vi "JSON Config Update Test Cases.vi"() -> ()   [LabVIEW 2021]
uses:
  OOB_Rx/CIFCoreOOB_Rx.lvclass/CIFCoreOOB_Rx.ctl
  <vilib>/CIF Foundation/CIF Out of Band Commands/CIFOutOfBand.lvclass/CIFOutOfBand.ctl
  OOB_Rx/Private/Command Settings.vi
  <vilib>/CIF Foundation/CIF Out of Band Commands/Accessors/Write Local OOB Data.vi
  <vilib>/CIF Foundation/CIF Out of Band Commands/Accessors/Read Local OOB Data.vi
  <vilib>/CIF Foundation/CIF Out of Band Commands/Read Commands.vi
  OOB_Rx/Private/Read Payload.vi
  <vilib>/CIF Foundation/CIF Out of Band Commands/Queue Command.vi
  <vilib>/CIF Foundation/CIF Out of Band Commands/Utilities/Command to Bitwise Command.vi
  OOB_Rx/CIFCoreOOB_Rx.lvclass
  C:/Program Files/National Instruments/LabVIEW 2021/vi.lib/CIF Foundation/CIF Out of Band Commands/CIFOutOfBand.lvclass
  <vilib>/CIF Foundation/CIF Out of Band Commands/Init OOB.vi
  <vilib>/addons/_JKI.lib/Serialization/JSON/Library/Unflatten From JSON String.vi
  <vilib>/addons/_JKI.lib/Serialization/JSON/JKI JSON Serialization.lvlib
  <vilib>/CIF Foundation/CIF Out of Band Commands/CIFOutOfBand.lvclass
panel:
  out "pass":bool
  out "error out":errorcluster
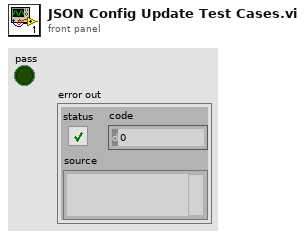
[diagram p1: front panel]
types:
  T1 = cluster{"Numeric":dbl, "String":string, "Boolean":bool}[]
  T2 = cluster{"Numeric":dbl, "Array":cluster{"Numeric":dbl, "String":string, "Boolean":bool}[], "string":string, "Null array":u8[]}
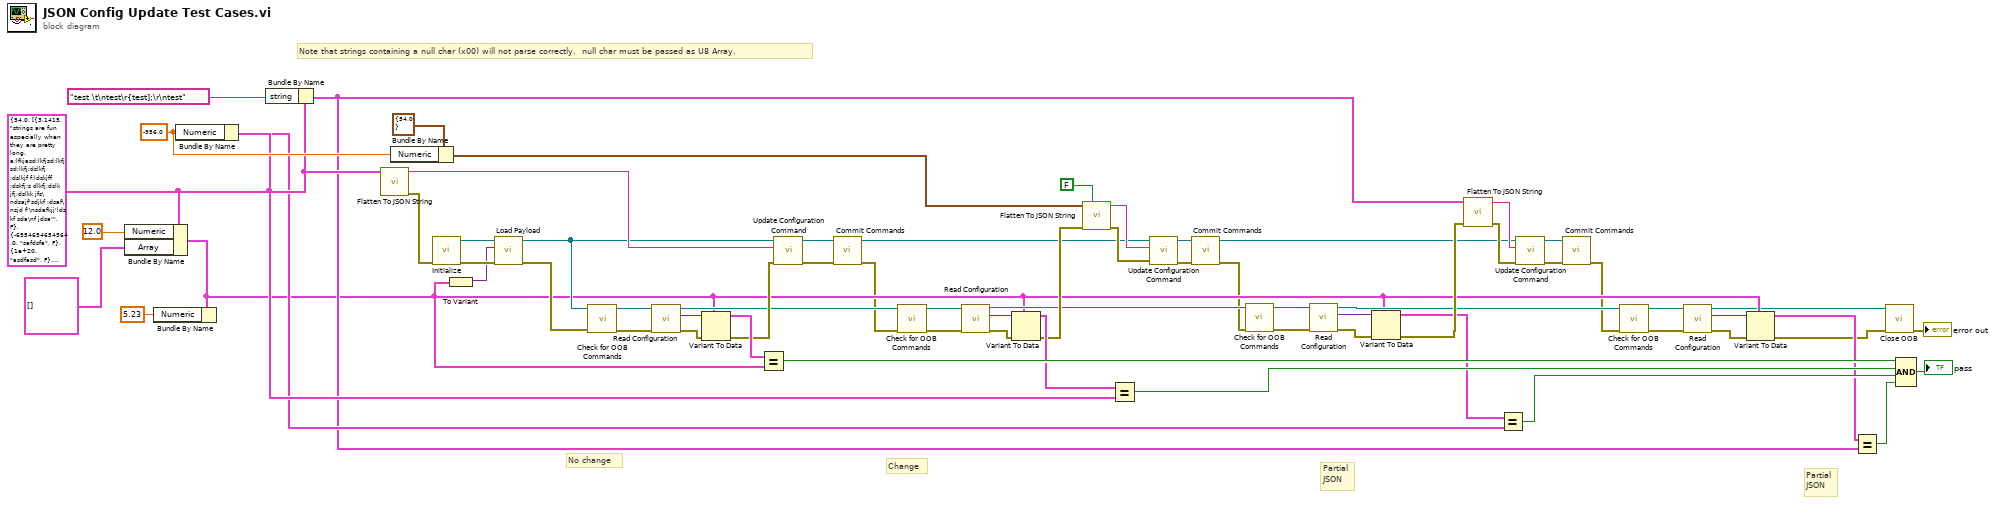
[diagram p0: block diagram]
diagram:
  w60 = -956.0 ("Numeric")
  w53 = T2 {"Numeric"=54.0, "Array"=[{"Numeric"=3.1415, "String"="strings are fun especially when they are pretty long. a;lfkjasd;lkfjsd;lkfjsd;lkfj;dslkfj ;dslkjf f;ldskjff ;dskfj;s dlkfj;dslk jfj;dslkk jfs\ndsajf'sdjkf ;dsaf\nsjd f'\nsdafkjj'lds kf sda\nf jdsa'", "Boolean"=FALSE}, {"Numeric"=-6554654654564.0, "String"="safdsfa", "Boolean"=FALSE}, {"Numeric"=1e+20, "String"="asdfasd", "Boolean"=FALSE}, {"Numeric"=2.0, "String"="afd", "Boolean"=TRUE}, {"Numeric"=12.34, "String"="data", "Boolean"=FALSE}], "string"="strings", "Null array"=[0]} ("Test Config")
  # "Note that strings containing a null char (x00) will not parse correctly.  null char must be passed as U8 Array."
  # "Partial\nJSON"
  # "Partial\nJSON"
  # "Change"
  # "No change"
  n1 = Bundle By Name(cluster=w53, "Numeric"=12.0, "Array"=T1 []) -> (w15:T2)
  n2 = Bundle By Name(cluster=w15, "Numeric"=5.23) -> ()  [unwired: 1 out]
  n3 = Bundle By Name(cluster=w53, "Numeric"=w60) -> (w52:T2)
  n4 = Bundle By Name(cluster=w53, "string"="test \t\ntest\r{test];\r\ntest" ("concatenated string")) -> (w49:T2)
  n5 = call <vilib>:"Flatten To JSON String.vi"("Variant"=w53) -> ("error out"=w64:errorcluster, "JSON String"=w66:string)  [unwired: 9 in]
  n6 = Bundle By Name(cluster=cluster{"Numeric":dbl} {"Numeric"=54.0} ("Test Config"), "Numeric"=w60) -> (w59:cluster{"Numeric":dbl})
  n7 = call "Initialize.vi"("error in"=w64) -> ("error out"=w45:errorcluster, "CoreOOB_Rx out"=w46:refnum<class "CIFCoreOOB_Rx.lvclass">)  [unwired: 9 in]
  n8 = To Variant(anything=w15) -> (Variant=w36:variant)
  n9 = call "Load Payload.vi"("error in (no error)"=w45, "Configuration Payload"=w36, "CoreOOB_Rx in"=w46) -> ("error out"=w44:errorcluster, "CoreOOB_Rx out"=w43:refnum<class "CIFCoreOOB_Rx.lvclass">)  [unwired: 7 in]
  n10 = call "Check for OOB Commands.vi"("error in (no error)"=w44, "CoreOOB_Rx in"=w43) -> ("error out"=w40:errorcluster, "CoreOOB_Rx out"=w41:refnum<class "CIFCoreOOB_Rx.lvclass">)  [unwired: 6 in, 2 out]
  n11 = call "Read Configuration.vi"("error in"=w40, "CoreOOB_Rx in"=w41) -> ("error out"=w38:errorcluster, "Configuration Data"=w39:variant, "CoreOOB_Rx out"=w30:refnum<class "CIFCoreOOB_Rx.lvclass">)  [unwired: 7 in]
  n12 = Variant To Data(error in=w38, type=w15, Variant=w39) -> (data=w37:T2, error out=w35:errorcluster)
  n13 = Equal?(x=w37, y=w15) -> (x = y?=w57:bool)
  n14 = call "Update Configuration Command.vi"("error in"=w35, "Config JSON"=w66, "CoreOOB_Rx in"=w43) -> ("error out"=w10:errorcluster, "CoreOOB_Rx out"=w11:refnum<class "CIFCoreOOB_Rx.lvclass">)  [unwired: 7 in]
  n15 = call <vilib>:"Commit Commands.vi"("error in"=w10, "OOB in"=w11) -> ("error out"=w9:errorcluster, "OOB out"=w8:refnum<class "CIFCoreOOB_Rx.lvclass">)  [unwired: 8 in]
  n16 = call "Check for OOB Commands.vi"("error in (no error)"=w9, "CoreOOB_Rx in"=w30) -> ("error out"=w32:errorcluster, "CoreOOB_Rx out"=w31:refnum<class "CIFCoreOOB_Rx.lvclass">)  [unwired: 6 in, 2 out]
  n17 = call "Read Configuration.vi"("error in"=w32, "CoreOOB_Rx in"=w31) -> ("error out"=w34:errorcluster, "Configuration Data"=w33:variant, "CoreOOB_Rx out"=w24:refnum<class "CIFCoreOOB_Rx.lvclass">)  [unwired: 7 in]
  n18 = Variant To Data(error in=w34, type=w15, Variant=w33) -> (data=w29:T2, error out=w28:errorcluster)
  n19 = call <vilib>:"Flatten To JSON String.vi"("Multiline (T)"=FALSE, "error in (no error)"=w28, "Variant"=w59) -> ("error out"=w58:errorcluster, "JSON String"=w62:string)  [unwired: 7 in]
  n20 = Equal?(x=w29, y=w53) -> (x = y?=w56:bool)
  n21 = call "Update Configuration Command.vi"("error in"=w58, "Config JSON"=w62, "CoreOOB_Rx in"=w8) -> ("error out"=w6:errorcluster, "CoreOOB_Rx out"=w7:refnum<class "CIFCoreOOB_Rx.lvclass">)  [unwired: 7 in]
  n22 = call <vilib>:"Commit Commands.vi"("error in"=w6, "OOB in"=w7) -> ("error out"=w5:errorcluster, "OOB out"=w4:refnum<class "CIFCoreOOB_Rx.lvclass">)  [unwired: 8 in]
  n23 = call "Check for OOB Commands.vi"("error in (no error)"=w5, "CoreOOB_Rx in"=w24) -> ("error out"=w27:errorcluster, "CoreOOB_Rx out"=w23:refnum<class "CIFCoreOOB_Rx.lvclass">)  [unwired: 6 in, 2 out]
  n24 = call "Read Configuration.vi"("error in"=w27, "CoreOOB_Rx in"=w23) -> ("error out"=w25:errorcluster, "Configuration Data"=w26:variant, "CoreOOB_Rx out"=w16:refnum<class "CIFCoreOOB_Rx.lvclass">)  [unwired: 7 in]
  n25 = Variant To Data(error in=w25, type=w15, Variant=w26) -> (data=w21:T2, error out=w22:errorcluster)
  n26 = call <vilib>:"Flatten To JSON String.vi"("error in (no error)"=w22, "Variant"=w49) -> ("error out"=w51:errorcluster, "JSON String"=w50:string)  [unwired: 8 in]
  n27 = Equal?(x=w21, y=w52) -> (x = y?=w55:bool)
  n28 = call "Update Configuration Command.vi"("error in"=w51, "Config JSON"=w50, "CoreOOB_Rx in"=w4) -> ("error out"=w2:errorcluster, "CoreOOB_Rx out"=w3:refnum<class "CIFCoreOOB_Rx.lvclass">)  [unwired: 7 in]
  n29 = call <vilib>:"Commit Commands.vi"("error in"=w2, "OOB in"=w3) -> ("error out"=w1:errorcluster)  [unwired: 8 in, 1 out]
  n30 = call "Check for OOB Commands.vi"("error in (no error)"=w1, "CoreOOB_Rx in"=w16) -> ("error out"=w17:errorcluster, "CoreOOB_Rx out"=w20:refnum<class "CIFCoreOOB_Rx.lvclass">)  [unwired: 6 in, 2 out]
  n31 = call "Read Configuration.vi"("error in"=w17, "CoreOOB_Rx in"=w20) -> ("error out"=w19:errorcluster, "Configuration Data"=w18:variant, "CoreOOB_Rx out"=w13:refnum<class "CIFCoreOOB_Rx.lvclass">)  [unwired: 7 in]
  n32 = Variant To Data(error in=w19, type=w15, Variant=w18) -> (data=w14:T2, error out=w12:errorcluster)
  n33 = Equal?(x=w14, y=w49) -> (x = y?=w48:bool)
  n34 = call <vilib>:"Close OOB.vi"("error in"=w12, "OOB in"=w13) -> ("error out"=→"error out":errorcluster)  [unwired: 9 in]
  n35 = Compound Arithmetic op=AND(w57, w56, w55, w48) -> (→"pass":bool)
